vi "rtout_discard.vi"(8 "error in":errorcluster, 11 "connection ID":refnum<k5>) -> (0 "error out":errorcluster, 3 "connection ID":refnum<k5>)   [LabVIEW 2016, in "AMC_VIs.lvlib"]
doc: "Discard all rtout value set by the set function(not applied yet)"
uses:
  AMC_VIs.lvlib
panel:
  out "params_cluster":cluster{"Numeric":i32}
  in  "Params_cluster":cluster{"Numeric":dbl}
  in  "results_cluster":cluster{"errNo":i32}
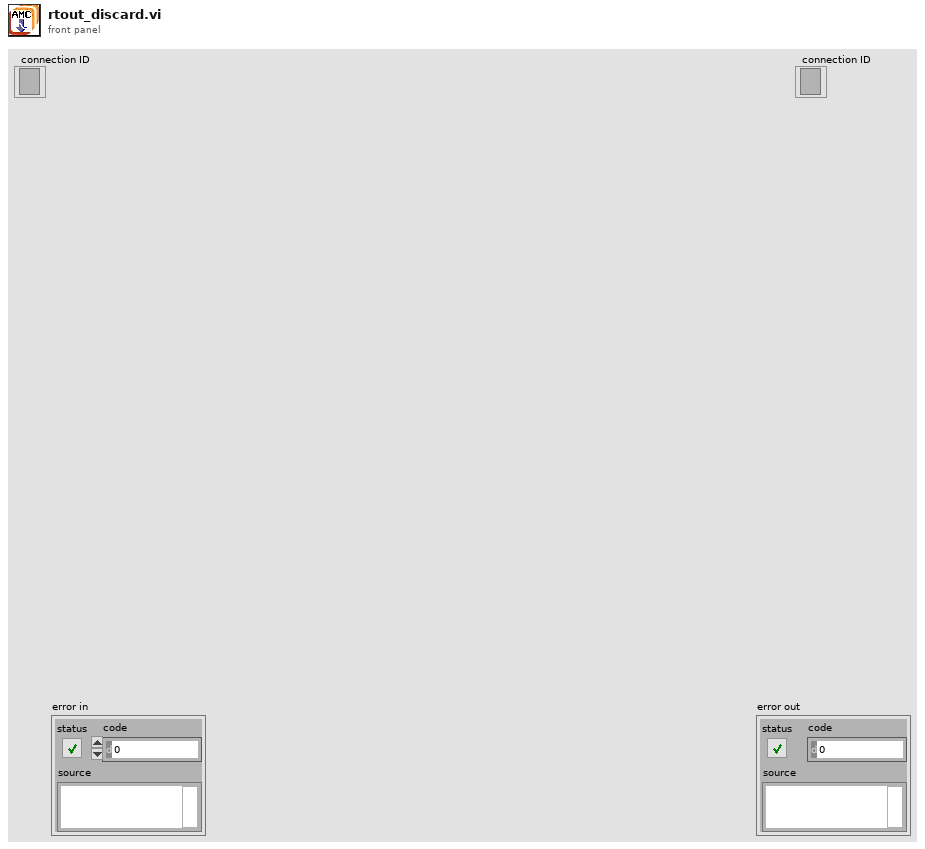
[diagram p1: front panel]
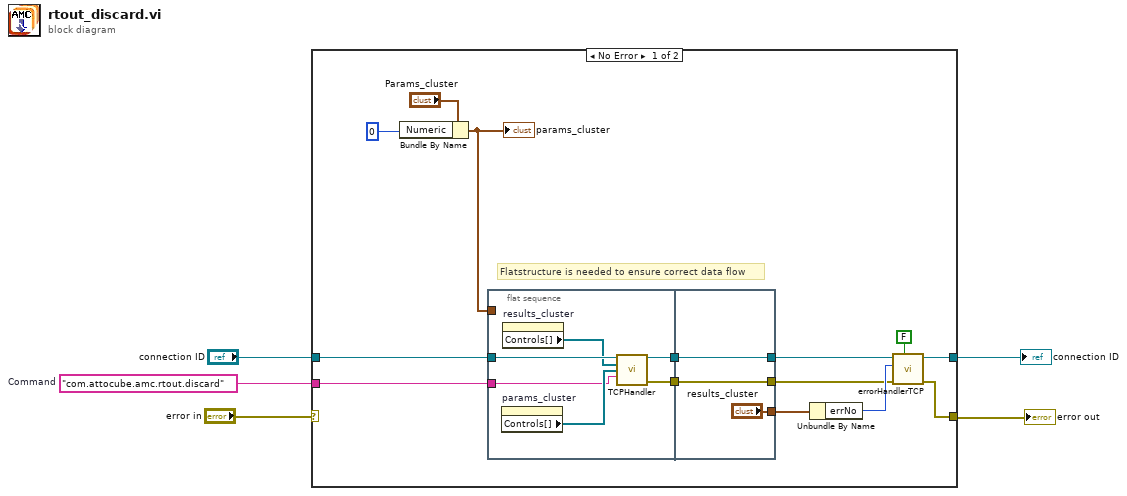
[diagram p0: block diagram]
diagram:
  w1 = "com.attocube.amc.rtout.discard"  # Command
  n1 = case shown="No Error" "error in" {
    selector: "error in" -> [_ w30]
    tunnel: [w17 w30] -> w5
    tunnel: [w19 w29] -> w4
    tunnel: "connection ID" -> [w16 w29]
    tunnel: w1 -> [w10 _]
    frame No Error {
      # "Flatstructure is needed to ensure correct data flow"
      n2 = Bundle By Name(cluster="Params_cluster", "Numeric"=0) -> (w7:cluster{"Numeric":dbl})
      "params_cluster" <- w7
      n3 = flat-sequence {
        tunnel: [w24] -> w12
        tunnel: w16 -> [w25]
        tunnel: w10 -> [w21]
        tunnel: [w20] -> w8
        tunnel: w7 -> [_]
        tunnel: ["results_cluster"] -> w13
        tunnel: [w28] -> w15
        tunnel: w12 -> [w28]
        tunnel: [w26] -> w9
        tunnel: w8 -> [w26]
        frame #0 {
          n4 = property on="params_cluster" class="Clust (strict)"() -> ("Controls[]"=w22:refnum<vi>[])  [unwired: 2 in, 2 out]
          n5 = property on="results_cluster" class="Clust (strict)"() -> ("Controls[]"=w23:refnum<vi>[])  [unwired: 2 in, 2 out]
          n6 = call "TCPHandler.vi"("connection ID"=w25, "results_cluster"=w23, "params_cluster"=w22, "method"=w21) -> ("connection ID"=w24:refnum<k5>, "error"=w20:errorcluster)  [unwired: 8 in, 2 out]
        }
        frame #1 {
        }
      }
      n7 = Unbundle By Name(w13) -> ("errNo"=w14:i32)
      n8 = call "errorHandlerTCP.vi"("show popup"=FALSE, "error in"=w9, "error number"=w14, "connection ID"=w15) -> ("error out"=w17:errorcluster, "connection ID"=w19:refnum<k5>)  [unwired: 6 in]
    }
    frame Error {
    }
  }
  "error out" <- w5
  "connection ID" <- w4
